vi "to string 3.1.vi"(8 "error in":errorcluster, 10 "data in":string, 11 "Shared Memory configuration in":refnum<class "Shared Memory configuration.lvclass">) -> (0 "error out":errorcluster, 2 "data out":string, 3 "Shared Memory configuration out":refnum<class "Shared Memory configuration.lvclass">)   [LabVIEW 2013, in "Shared Memory configuration.lvclass"]
uses:
  Shared Memory configuration.lvclass
  Shared Memory configuration.lvclass/Shared Memory configuration.ctl
  <vilib>/NI/Configuration Framework/serializable configuration/NISE_CEF_serializable configuration.lvclass
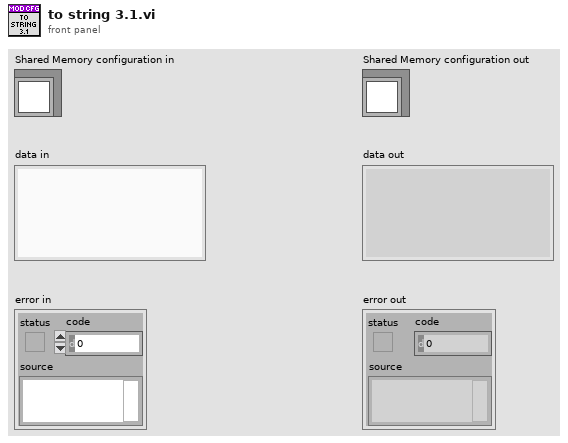
[diagram p1: front panel]
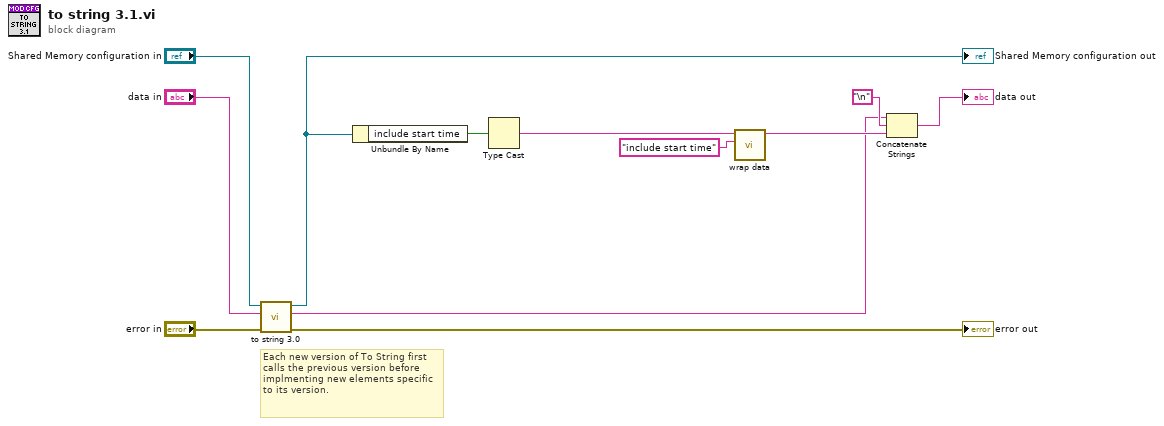
[diagram p0: block diagram]
diagram:
  # "Each new version of To String first calls the previous version before implmenting new elements specific to its version."
  n1 = call "to string 3.0.vi"("error in"="error in", "data in"="data in", "Shared Memory configuration in"="Shared Memory configuration in") -> ("error out"=→"error out":errorcluster, "data out"=w1:string, "Shared Memory configuration out"=w4:refnum<class "Shared Memory configuration.lvclass">)  [unwired: 6 in]
  "Shared Memory configuration out" <- w4
  n2 = Unbundle By Name(w4) -> ("include start time"=w8:bool)
  n3 = Type Cast(x=w8) -> (*(type *) &x=w7:string)  [unwired: 1 in]
  n4 = call <vilib>:"wrap data.vi"("identifier"="include start time", "data to wrap"=w7) -> ("wrapped data"=w9:string)  [unwired: 9 in]
  n5 = Concatenate Strings(w1, "\n", w9) -> (→"data out":string)
